vi "Receiver.vi"() -> ()   [LabVIEW 2015]
uses:
  <instrlib>/niUSRP/niUSRP Fetch Rx Data (CDB WDT).vi
  <vilib>/measure/maspectr.llb/FFT Power Spectrum and PSD for 1 Chan (CDB).vi
  <vilib>/Analysis/NI_AALPro.lvlib
  <vilib>/measure/NI_MAPro.lvlib
panel:
  out "Waveform Graph 2":cluster{"f0":dbl, "df":dbl, "magnitude":dbl[]}(graph)
  out "Waveform Graph":waveform(dbl)[](graph)
  out "error out":errorcluster
  out "coerced gain":dbl format="%#_6f"
  out "coerced carrier\n frequency":dbl=100000.0 format="%#_6p"
  out "coerced IQ rate":dbl=100000.0 format="%#_6p"
  in  "number of samples":i64=1000
  in  "carrier frequency":dbl=100000.0 format="%#_6p"
  in  "device names":refnum<k15>
  in  "IQ rate":dbl=100000.0 format="%#_6p"
  in  "gain":dbl format="%#_6f"
  in  "active antenna":string
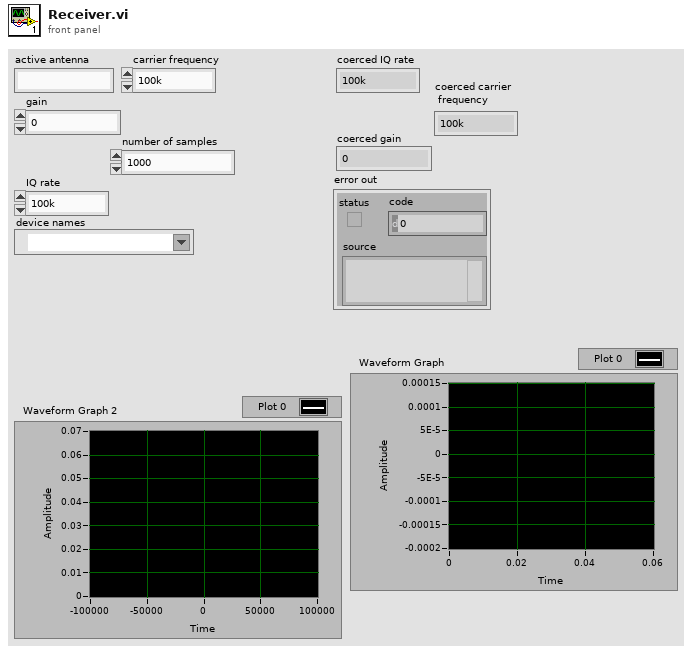
[diagram p1: front panel]
types:
  T1 = typedef "Sound Output Task ID.ctl" = u32
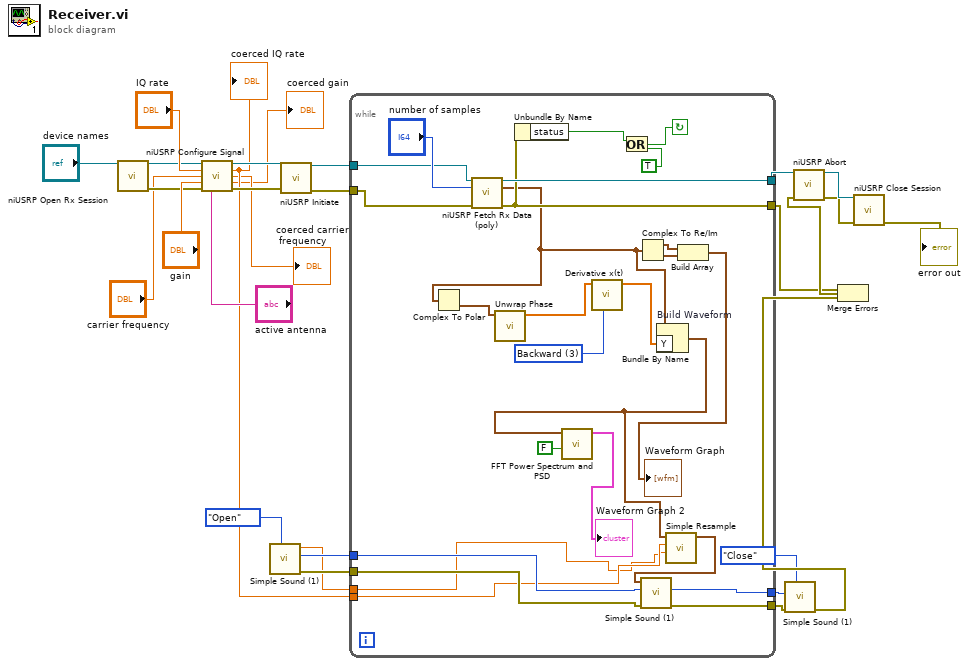
[diagram p0: block diagram]
diagram:
  n1 = call <instrlib>:"niUSRP Open Rx Session.vi"("device names"="device names") -> ("session handle out"=w25:refnum<k15>, "error out"=w23:errorcluster)  [unwired: 13 in]
  n2 = call <instrlib>:"niUSRP Configure Signal.vi"("session handle"=w25, "IQ rate"="IQ rate", "carrier frequency"="carrier frequency", "gain"="gain", "error in (no error)"=w23, "active antenna"="active antenna") -> ("session handle out"=w21:refnum<k15>, "coerced IQ rate"=w12:dbl, "coerced carrier frequency"=→"coerced carrier\n frequency":dbl, "coerced gain"=→"coerced gain":dbl, "error out"=w22:errorcluster)  [unwired: 5 in]
  "coerced IQ rate" <- w12
  n3 = call "Simple Sound (1).vi"("Action"=enum16{"Open", "Write", "Close"}."Open") -> ("error out"=w7:errorcluster, "task ID out"=w8:T1, "sample rate (S/s)"=w2:dbl)  [unwired: 6 in]
  n4 = call <instrlib>:"niUSRP Initiate.vi"("session handle"=w21, "error in (no error)"=w22) -> ("session handle out"=w19:refnum<k15>, "error out"=w18:errorcluster)  [unwired: 12 in]
  n5 = while {
    tunnel: w19 -> [w51]
    tunnel: w18 -> [w53]
    tunnel: [w49] -> w13
    tunnel: [w50] -> w15
    tunnel: w12 -> [w32]
    tunnel: w8 -> [w37]
    tunnel: w7 -> [w36]
    tunnel: [w35] -> w6
    tunnel: [w34] -> w5
    tunnel: w2 -> [w31]
    stop <- w52 continue-if-true
    w33 = u16 3 items=["2nd Order Central", "4th Order Central", "Forward", "Backward"] ("method")
    n6 = call-poly <instrlib>:"niUSRP Fetch Rx Data (poly).vi"("session handle"=w51, "number of samples"="number of samples", "error in (no error)"=w53) -> ("session handle out"=w50:refnum<k15>, "data"=w44:waveform(cdb), "error out"=w49:errorcluster)  [unwired: 9 in, 1 out]
    n7 = Complex To Polar(r * e^(i*theta)=w44) -> (theta=w47:waveform(dbl))  [unwired: 1 out]
    n8 = call <vilib>:"Unwrap Phase.vi"("Phase"=w47) -> ("Unwrapped Phase"=w46:dbl[])  [unwired: 9 in, 1 out]
    n9 = Unbundle By Name(w49) -> ("status"=w48:bool)
    n10 = call <vilib>:"Derivative x(t).vi"("method"=w33, "X"=w46) -> ("dX/dt"=w45:dbl[])  [unwired: 8 in, 1 out]
    n11 = Or(x=w48, y=TRUE) -> (x .or. y?=w52:bool)
    n12 = Complex To Re/Im(x + iy=w44) -> (x=w43:waveform(dbl), y=w42:waveform(dbl))
    n13 = Bundle By Name "Build Waveform"(cluster=w44, "Y"=w45) -> (w39:waveform(cdb))
    n14 = call-poly <vilib>:"FFT Power Spectrum and PSD.vi"("dB On (F)"=FALSE, "time signal"=w39) -> ("Power Spectrum / PSD"=→"Waveform Graph 2":cluster{"f0":dbl, "df":dbl, "magnitude":dbl[]})  [unwired: 6 in, 3 out]
    n15 = call "Simple Resample.vi"("sample rate (S/s)"=w31, "coerced IQ Rate"=w32, "input waveform"=w39) -> ("output waveform"=w38:waveform(dbl))  [unwired: 8 in]
    n16 = call "Simple Sound (1).vi"("error in"=w36, "task ID"=w37, "data"=w38) -> ("error out"=w35:errorcluster, "task ID out"=w34:T1)  [unwired: 4 in, 1 out]
    n17 = Build Array(w43, w42) -> (→"Waveform Graph":waveform(dbl)[])
  }
  n18 = call "Simple Sound (1).vi"("Action"=enum16{"Open", "Write", "Close"}."Close", "error in"=w6, "task ID"=w5) -> ("error out"=w4:errorcluster)  [unwired: 4 in, 2 out]
  n19 = Merge Errors "Merge Errors"(w13, w4) -> (w14:errorcluster)
  n20 = call <instrlib>:"niUSRP Abort.vi"("session handle"=w15, "error in (no error)"=w14) -> ("session handle out"=w17:refnum<k15>, "error out"=w16:errorcluster)  [unwired: 12 in]
  n21 = call <instrlib>:"niUSRP Close Session.vi"("session handle"=w17, "error in (no error)"=w16) -> ("error out"=→"error out":errorcluster)  [unwired: 13 in]
